vi "StopZ.vi"(10 "Optciones":bool[](array[boolean])) -> (2 "parar":bool)   [LabVIEW 2018]
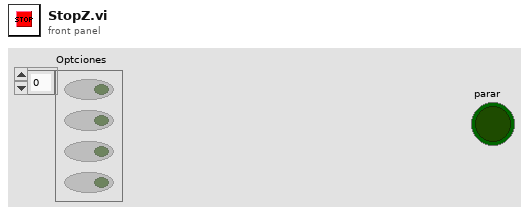
[diagram p1: front panel]
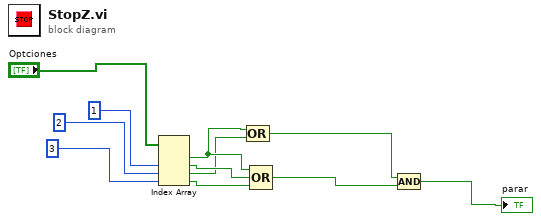
[diagram p0: block diagram]
diagram:
  n1 = Index Array(array="Optciones", index #2=1 ("index"), index #3=2 ("index"), index #4=3 ("index")) -> (element #1=w7:bool, element #2=w6:bool, element #3=w5:bool, element #4=w1:bool)  [unwired: 1 in]
  n2 = Compound Arithmetic op=OR(w7, w5) -> (w4:bool)
  n3 = Compound Arithmetic op=OR(w7, w6, w1) -> (w3:bool)
  n4 = Compound Arithmetic op=AND(w4, w3) -> (→"parar":bool)
